vi "Read Old.vi"(8 "Error In":errorcluster, 11 "Set Delimiter In":refnum<class "SetDelimiter.lvclass">) -> (0 "Error Out":errorcluster, 2 "Old Value":T1, 3 "Set Delimiter Out":refnum<class "SetDelimiter.lvclass">)   [LabVIEW 2018, in "Toolkit.lvlib" / "Tokens.lvlib" / "SetDelimiter.lvclass"]
uses:
  SetDelimiter.lvclass
  Type Definitions/Delimiters.ctl
  Toolkit.lvlib
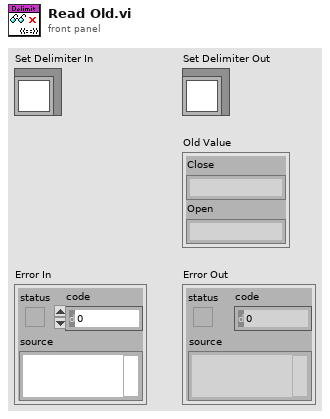
[diagram p1: front panel]
types:
  T1 = typedef "Toolkit.lvlib/Delimiters.ctl" = cluster{"Close":string, "Open":string}
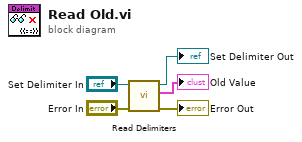
[diagram p0: block diagram]
diagram:
  n1 = call-dynamic "Read Delimiters.vi"("Error In"="Error In", "Token In"="Set Delimiter In") -> ("Error Out"=→"Error Out":errorcluster, "Delimiters"=→"Old Value":T1, "Token Out"=→"Set Delimiter Out":refnum<class "SetDelimiter.lvclass">)  [unwired: 7 in]
